vi "Unregister (async).vi"(8 "error in (no error)":errorcluster, 10 "Endpoint URI":string, 11 "WAMP Client in":refnum<class "WAMP Client.lvclass">) -> (0 "error out":errorcluster, 2 "notifier out":refnum<notifier>, 3 "WAMP Client out":refnum<class "WAMP Client.lvclass">)   [LabVIEW 2020, in "wamplv.lvlib" / "WAMP Client.lvclass"]
uses:
  WAMP Client.lvclass
  TypeDef/Internal Message Type.ctl
  API/TypeDefs/WAMP error.ctl
  API/TypeDefs/Combined error.ctl
  TypeDef/Success or error.ctl
  TypeDef/Unregister request.ctl
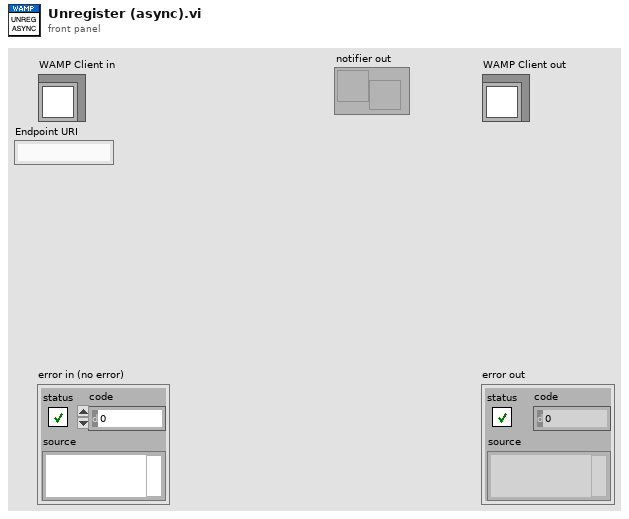
[diagram p1: front panel]
types:
  T1 = typedef "wamplv.lvlib/WAMP Client.lvclass/Unregister request.ctl" = cluster{"URI":string, "Unregister result notifier":refnum<notifier>}
  T2 = typedef "wamplv.lvlib/WAMP Client.lvclass/Success or error.ctl" = cluster{"Success?":bool, "URI":string, "Combined Error":T3}
  T3 = typedef "wamplv.lvlib/WAMP Client.lvclass/Combined error.ctl" = cluster{"Error?":bool, "WAMP Error":T4, "Error":errorcluster}
  T4 = typedef "wamplv.lvlib/WAMP Client.lvclass/WAMP error.ctl" = cluster{"Details":string, "ArgumentKw Payload":string, "Error?":bool, "Error URI":string, "Arguments Payload":string}
  T5 = typedef "wamplv.lvlib/WAMP Client.lvclass/Internal Message Type.ctl" = enum16{"Subscribe", "Handle Subscribed", "Handle Event", "Unsubscribe", "Handle Unsubscribed", "Publish", "Handled Published", "Goodbye", "Handle Goodbye", "Call", "Handle Result", "Register", "Handle Registered", "Unregister", "Handle Unregistered", "Handle Invocation", "Yield", "Error"}
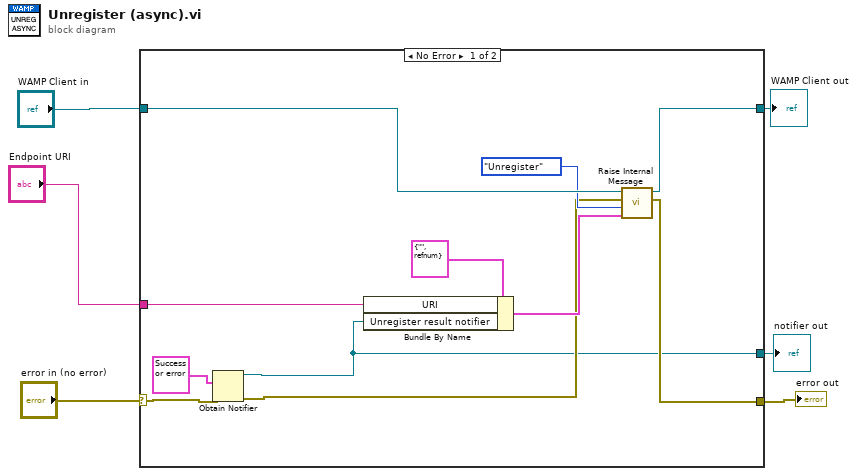
[diagram p0: block diagram]
diagram:
  n1 = case shown="No Error" "error in (no error)" {
    selector: "error in (no error)" -> [w10 w19]
    tunnel: [w12 w19] -> w5
    tunnel: [w11 w18] -> w3
    tunnel: "WAMP Client in" -> [w17 w18]
    tunnel: [w8 _] -> w1
    tunnel: "Endpoint URI" -> [w15 _]
    frame No Error {
      n2 = Obtain Notifier(notification data type=T2 {"Success?"=FALSE, "URI"="", "Combined Error"={"Error?"=FALSE, "WAMP Error"={"Details"="{}", "ArgumentKw Payload"="{}", "Error?"=FALSE, "Error URI"="", "Arguments Payload"=""}, "Error"={"status"=FALSE, "code"=0, "source"=""}}} ("Sucess or error"), error in (no error)=w10) -> (notifier out=w8:refnum<notifier>, error out=w9:errorcluster)  [unwired: 2 in, 1 out]
      n3 = Bundle By Name(cluster=T1 {"URI"="", "Unregister result notifier"=refnum} ("Unregister Request"), "URI"=w15, "Unregister result notifier"=w8) -> (w16:T1)
      n4 = call-dynamic "Raise Internal Message.vi"("Variant"=w16, "Internal Message Type"=Internal_Message_Type."Unregister", "error in (no error)"=w9, "WAMP Client in"=w17) -> ("error out"=w12:errorcluster, "WAMP Client out"=w11:refnum<class "WAMP Client.lvclass">)  [unwired: 6 in]
    }
    frame Error {
    }
  }
  "error out" <- w5
  "WAMP Client out" <- w3
  "notifier out" <- w1
